vi "measconfig read file.vi"(8 "error in (no error)":errorcluster, 11 "measurement file":path) -> (0 "error out":errorcluster, 3 "measurements":T1[](array[typedef]))   [LabVIEW 2013]
uses:
  measconfig cluster.ctl
  measurement sweep parameter.ctl
  devices/magnet/magnet polar field.ctl
  <vilib>/Utility/config.llb/NI_LVConfig.lvlib
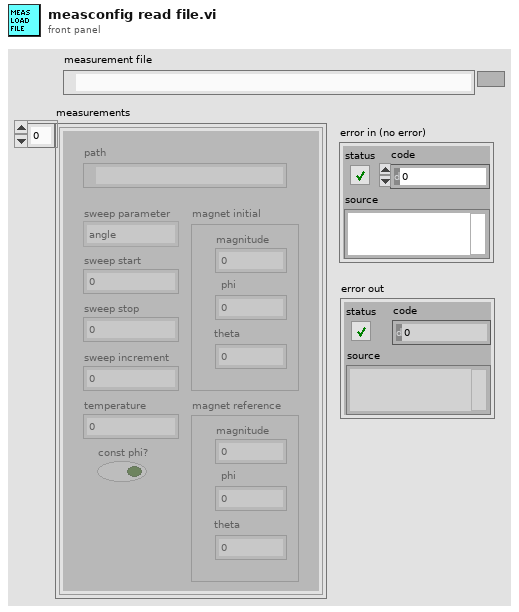
[diagram p1: front panel]
types:
  T1 = typedef "measconfig cluster.ctl" = cluster{"sweep parameter":T2, "sweep start":dbl, "sweep stop":dbl, "sweep increment":dbl, "temperature":dbl, "path":path, "magnet initial":T3, "magnet reference":T3, "const phi?":bool}
  T2 = typedef "measurement sweep parameter.ctl" = enum16{"angle", "magnetic field"}
  T3 = typedef "magnet polar field.ctl" = cluster{"magnitude":dbl, "phi":dbl, "theta":dbl}
  T4 = typedef "NI_LVConfig.lvlib/Config Data RefNum.ctl" = refnum<k1>
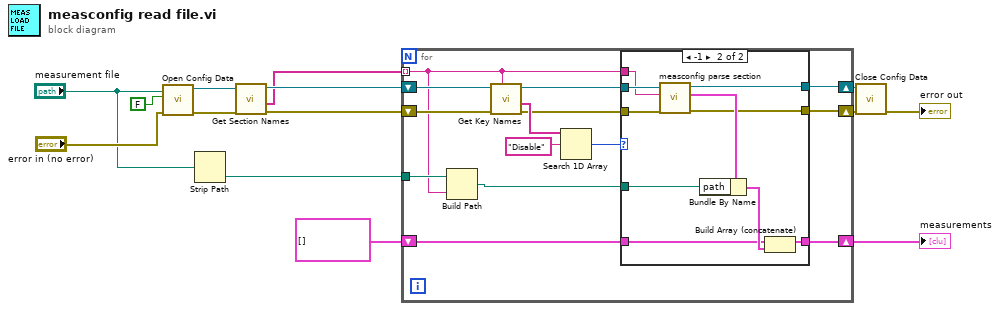
[diagram p0: block diagram]
diagram:
  n1 = call <vilib>:"Open Config Data.vi"("error in (no error)"="error in (no error)", "create file if necessary (T)"=FALSE, "configuration file path"="measurement file") -> ("error out"=w11:errorcluster, "refnum"=w12:T4)  [unwired: 6 in, 1 out]
  n2 = Strip Path(path="measurement file") -> (stripped path=w3:path)  [unwired: 1 out]
  n3 = call <vilib>:"Get Section Names.vi"("error in (no error)"=w11, "refnum"=w12) -> ("error out"=w9:errorcluster, "section names"=w5:string[], "refnum out"=w10:T4)  [unwired: 7 in]
  n4 = for {
    tunnel: w5 -> [w15] mode=indexing
    shift-right: [w21] -> w7
    shift-left: w10 -> [w28]
    shift-right: [w20] -> w8
    shift-left: w9 -> [w27]
    shift-right: [w17] -> w1
    shift-left: T1[] [] ("measurements") -> [w16]
    tunnel: w3 -> [w19]
    n5 = Build Path(base path=w19, name or relative path=w15) -> (appended path=w18:path)
    n6 = call <vilib>:"Get Key Names.vi"("section"=w15, "error in (no error)"=w27, "refnum"=w28) -> ("error out"=w22:errorcluster, "key names"=w26:string[], "refnum out"=w23:T4)  [unwired: 5 in, 1 out]
    n7 = Search 1D Array(1D array=w26, element="Disable") -> (index of element=w24:i32)  [unwired: 1 in]
    n8 = case shown="-1" w24 {
      tunnel: w23 -> [w31 w40]
      tunnel: w22 -> [w30 w39]
      tunnel: w15 -> [_ w38]
      tunnel: [w31 w37] -> w21
      tunnel: [w30 w36] -> w20
      tunnel: w18 -> [_ w35]
      tunnel: w16 -> [w29 w32]
      tunnel: [w29 w33] -> w17
      frame 0, Default {
      }
      frame -1 {
        n9 = call "measconfig parse section.vi"("error in (no error)"=w39, "section name"=w38, "refnum"=w40) -> ("error out"=w36:errorcluster, "measurement definition"=w41:T1, "refnum out"=w37:T4)  [unwired: 6 in]
        n10 = Bundle By Name(cluster=w41, "path"=w35) -> (w34:T1)
        n11 = Build Array (concatenate)(w32, w34) -> (w33:T1[])
      }
    }
  }
  "measurements" <- w1
  n12 = call <vilib>:"Close Config Data.vi"("error in (no error)"=w8, "refnum"=w7) -> ("error out"=→"error out":errorcluster)  [unwired: 8 in, 1 out]
